vi "Delete Mapping.vi"(8 "error in (no error)":errorcluster, 9 "row name":string, 10 "scale index":i32, 11 "Scaling configuration in":refnum<class "Scaling configuration.lvclass">) -> (0 "error out":errorcluster, 3 "Scaling configuration out":refnum<class "Scaling configuration.lvclass">)   [LabVIEW 2013, in "Scaling configuration.lvclass"]
uses:
  Scaling configuration.lvclass
  Scaling configuration.lvclass/Scaling configuration.ctl
  <vilib>/NI/Tag Bus/tag/tag descriptor.lvclass/tag descriptor.ctl
  <vilib>/NI/Tag Bus/tag/tag descriptor.lvclass
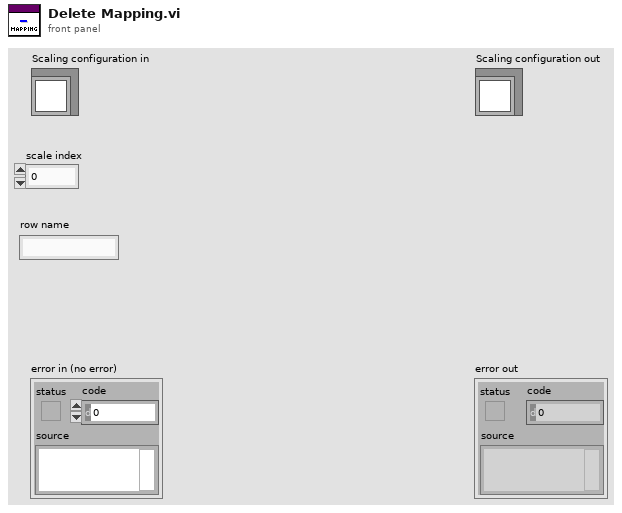
[diagram p1: front panel]
types:
  T1 = typedef "Scaling configuration.lvclass/scale data types.ctl" = enum16{"Double", "Single", "I64", "I32", "I16", "I8", "U64", "U32", "U16", "U8"}
  T2 = cluster{"mappings":cluster{"input channel":refnum<class "TBM channel.lvclass">, "output channel":refnum<class "TBM channel.lvclass">, "input data type":T1, "output data type":T1}[], "name":string}[]
  T3 = cluster{"mappings":cluster{"input channel":refnum<class "TBM channel.lvclass">, "output channel":refnum<class "TBM channel.lvclass">, "input data type":T1, "output data type":T1}[], "name":string}
  T4 = cluster{"input channel":refnum<class "TBM channel.lvclass">, "output channel":refnum<class "TBM channel.lvclass">, "input data type":T1, "output data type":T1}[]
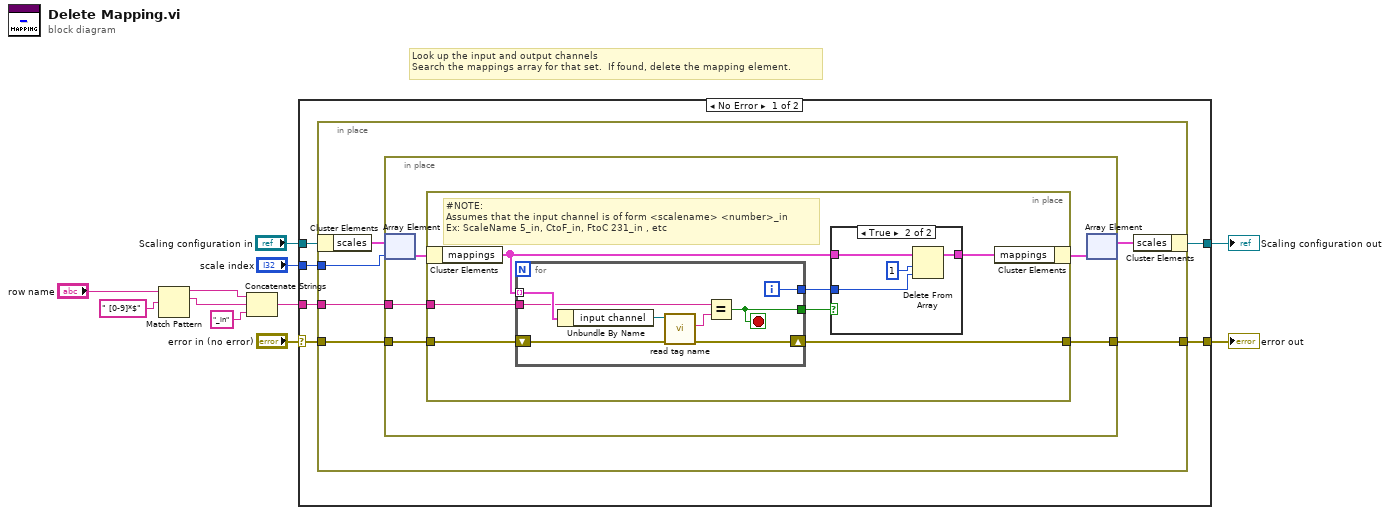
[diagram p0: block diagram]
diagram:
  # "Look up the input and output channels\nSearch the mappings array for that set.  If found, delete the mapping element."
  n1 = Match Pattern(string="row name", regular expression=" [0-9]*$") -> (before substring=w5:string, match substring=w2:string)  [unwired: 1 in, 2 out]
  n2 = Concatenate Strings(w5, w2, "_in" ("string")) -> (w3:string)
  n3 = case shown="No Error" "error in (no error)" {
    selector: "error in (no error)" -> [w15 w50]
    tunnel: [w14 w50] -> w10
    tunnel: [w17 w49] -> w8
    tunnel: "Scaling configuration in" -> [w12 w49]
    tunnel: "scale index" -> [w16 _]
    tunnel: w3 -> [w13 _]
    frame No Error {
      n4 = in-place {
        in-place-border: w16 -> [w22]
        in-place-border: w15 -> [w20]
        in-place-border: [w19] -> w14
        in-place-border: w13 -> [w18]
        n5 = in-place-cluster #1(w12) -> ("scales"=w23:T2)
        n6 = in-place {
          in-place-border: w20 -> [w26]
          in-place-border: [w25] -> w19
          in-place-border: w18 -> [w24]
          n7 = in-place-array #2(w23, w22) -> (w28:T3)
          n8 = in-place {
            in-place-border: w26 -> [w33]
            in-place-border: [w32] -> w25
            in-place-border: w24 -> [w31]
            # "#NOTE:\nAssumes that the input channel is of form <scalename> <number>_in\nEx: ScaleName 5_in, CtoF_in, FtoC 231_in , etc"
            n9 = in-place-cluster #3(w28) -> ("mappings"=w35:T4)
            n10 = for {
              tunnel: w35 -> [w48] mode=indexing
              tunnel: w31 -> [w45]
              tunnel: [w44] -> w30
              tunnel: [w43] -> w29
              shift-right: [w41] -> w32
              shift-left: w33 -> [w42]
              i -> [w43]
              stop <- w44 stop-if-true
              n11 = Unbundle By Name(w48) -> ("input channel"=w47:refnum<class "TBM channel.lvclass">)
              n12 = call <vilib>:"read tag name.vi"("error in"=w42, "system tag in"=w47) -> ("error out"=w41:errorcluster, "name"=w46:string)  [unwired: 7 in, 1 out]
              n13 = Equal?(x=w45, y=w46) -> (x = y?=w44:bool)
            }
            n14 = case shown="True" w30 {
              tunnel: w35 -> [w36 w40]
              tunnel: w29 -> [_ w38]
              tunnel: [w36 w37] -> w34
              frame False {
              }
              frame True {
                n15 = Delete From Array(array=w40, length=1, index=w38) -> (array with subset deleted=w37:T4)  [unwired: 1 out]
              }
            }
            n16 = in-place-cluster #3("mappings"=w34) -> (w27:T3)
          }
          n17 = in-place-array #2(w27) -> (w21:T2)  [unwired: 1 out]
        }
        n18 = in-place-cluster #1("scales"=w21) -> (w17:refnum<class "Scaling configuration.lvclass">)
      }
    }
    frame Error {
    }
  }
  "error out" <- w10
  "Scaling configuration out" <- w8
